vi "startMeasurement.vi"(6 "MeasConfigType":T1, 7 "Device Handle":i32, 8 "error in (no error)":errorcluster, 9 "NumOfScans":i16, 10 "a_hWnd":i32, 11 "SEDSpectrometer in":refnum<class "FiberSpectrograph.lvclass">) -> (0 "error out":errorcluster, 1 "StartTime":u32, 2 "Status":string, 3 "SEDSpectrometer out":refnum<class "FiberSpectrograph.lvclass">)   [LabVIEW 2016, in "FiberSpectrograph.lvclass"]
uses:
  FiberSpectrograph.lvclass
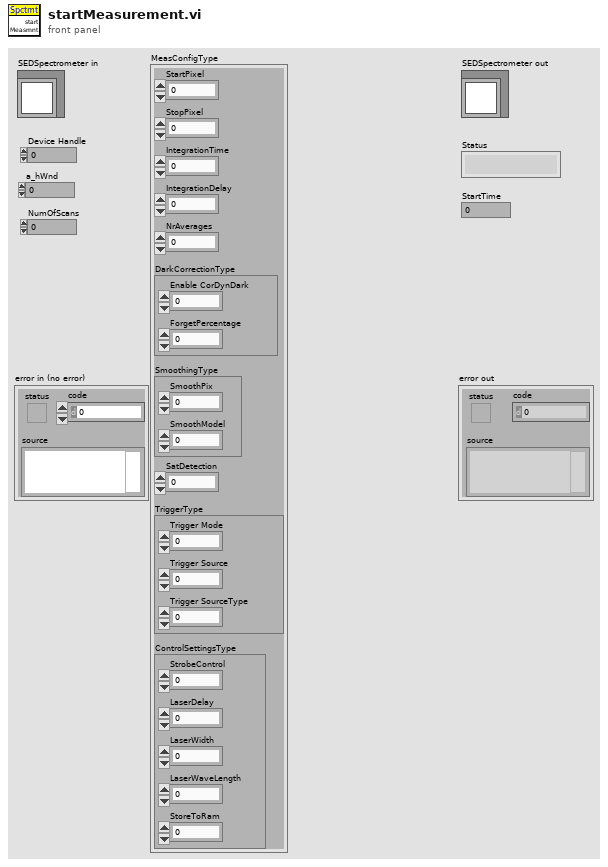
[diagram p1: front panel]
types:
  T1 = cluster{"StartPixel":u16, "StopPixel":u16, "IntegrationTime":sgl, "IntegrationDelay":u32, "NrAverages":u32, "DarkCorrectionType":cluster{"Enable CorDynDark":u8, "ForgetPercentage":u8}, "SmoothingType":cluster{"SmoothPix":u16, "SmoothModel":u8}, "SatDetection":u8, "TriggerType":cluster{"Trigger Mode":u8, "Trigger Source":u8, "Trigger SourceType":u8}, "ControlSettingsType":cluster{"StrobeControl":u16, "LaserDelay":u32, "LaserWidth":u32, "LaserWaveLength":sgl, "StoreToRam":u16}}
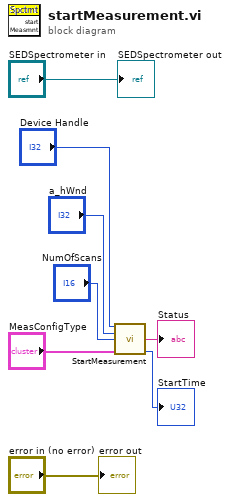
[diagram p0: block diagram]
diagram:
  n1 = call "StartMeasurement.vi"("a_hDevice"="Device Handle", "a_hWnd"="a_hWnd", "a_Nmsr"="NumOfScans", "MeasConfigType"="MeasConfigType") -> ("Status"=→"Status":string, "StartTime"=→"StartTime":u32)  [unwired: 10 in]
  "error out" <- "error in (no error)"
  "SEDSpectrometer out" <- "SEDSpectrometer in"
